vi "Assert Equal JSON.vi"(7 "Label":string, 8 "error in (no error)":errorcluster, 10 "JSON String Y":string, 11 "JSON String X":string) -> (0 "error out":errorcluster)   [LabVIEW 2020, in "TEST - JKI JSON Object Serialization.lvlib"]
uses:
  tests/TEST - JKI JSON Object Serialization.lvlib
  <vilib>/addons/_JKI Toolkits/Caraya/classes/Assert/Assert Equal Value_Variant.vi
  <vilib>/addons/_JKI Toolkits/Caraya/classes/Assert/Assert.lvclass
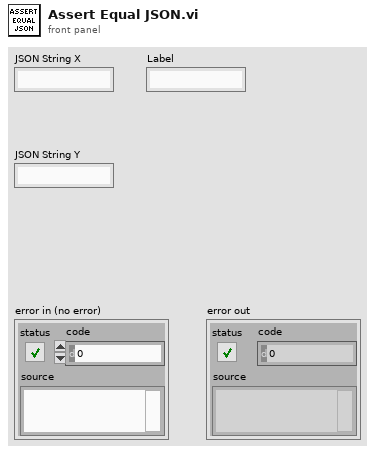
[diagram p1: front panel]
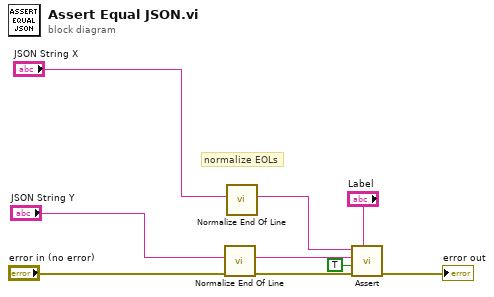
[diagram p0: block diagram]
diagram:
  # "normalize EOLs"
  n1 = call <vilib>:"Normalize End Of Line.vi"("string in"="JSON String Y") -> ("string out"=w8:string)  [unwired: 7 in]
  n2 = call <vilib>:"Normalize End Of Line.vi"("string in"="JSON String X") -> ("string out"=w7:string)  [unwired: 7 in]
  n3 = call-poly <vilib>:"Assert.vi"("Label"="Label", "error in (no error)"="error in (no error)", "Register with caller test (F)"=TRUE, "Y"=w8, "X"=w7) -> ("error out"=→"error out":errorcluster)  [unwired: 5 in, 1 out]
